vi "Find Unique Zero.vi"(7 "VI in":refnum<vi>, 8 "Error In":errorcluster, 9 "Zero Finder Parameters":T1, 10 "max tau":dbl, 11 "Zeros":dbl[](array[numeric])) -> (0 "Error Out":errorcluster, 3 "Phase Lifetime":dbl)   [LabVIEW 2019]
uses:
  tau_phi & tau_m Zero Finder Parameters.ctl
  <vilib>/gmath/NI_Gmath.lvlib
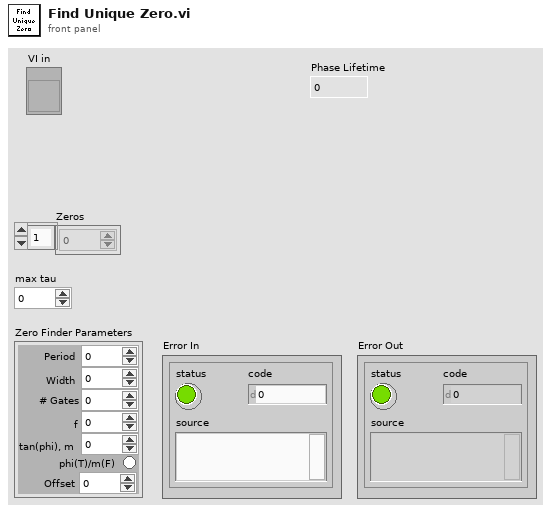
[diagram p1: front panel]
types:
  T1 = typedef "tau_phi & tau_m Zero Finder Parameters.ctl" = cluster{"Period":ext, "Width":ext, "# Gates":ext, "f":ext, "tan(phi), m":ext, "phi(T)/m(F)":bool, "Offset":ext}
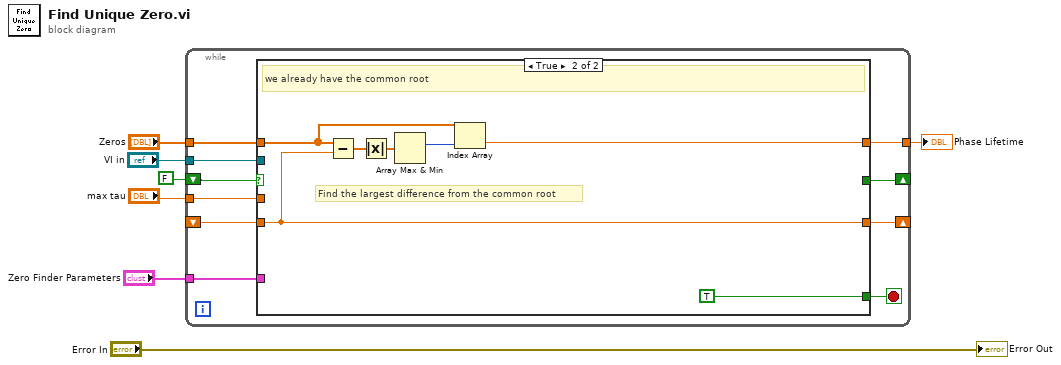
[diagram p0: block diagram]
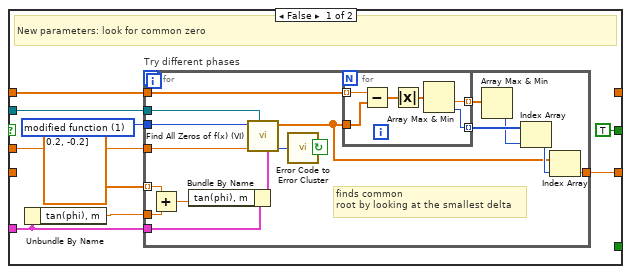
[diagram p2: hidden frame]
diagram:
  n1 = while {
    tunnel: "Zero Finder Parameters" -> [w13]
    shift-right: [w14] -> _
    shift-left: _ -> [w16]
    tunnel: "Zeros" -> [w17]
    tunnel: [w15] -> w4
    tunnel: "VI in" -> [w12]
    tunnel: "max tau" -> [w11]
    shift-right: [w8] -> _
    shift-left: FALSE -> [w9]
    stop <- w10 stop-if-true
    n2 = case shown="True" w9 {
      tunnel: w17 -> [w20 w51]
      tunnel: w16 -> [_ w55]
      tunnel: [_ w50] -> w15
      tunnel: [w19 w55] -> w14
      tunnel: w13 -> [w21 _]
      tunnel: w12 -> [w24 _]
      tunnel: w11 -> [w22 _]
      tunnel: [_ TRUE] -> w10
      tunnel: [TRUE _] -> w8
      frame False {
        w23 = u16 1 items=["fixed function", "modified function"] ("step type")
        # "New parameters: look for common zero"
        n3 = Unbundle By Name(w21) -> ("tan(phi), m"=w26:ext)
        n4 = for "Try different phases" {
          tunnel: w26 -> [w43]
          tunnel: dbl[] [0.1, -0.1, 0.2, -0.2] ("x") -> [w42] mode=indexing
          tunnel: w24 -> [w41]
          tunnel: w23 -> [w40]
          tunnel: w22 -> [w39]
          tunnel: w21 -> [w38]
          tunnel: w20 -> [w33]
          tunnel: [w27] -> w19
          stop <- w34 continue-if-true
          # "finds common\nroot by looking at the smallest delta"
          n5 = Add(x=w42, y=w43) -> (x+y=w36:ext)
          n6 = Bundle By Name(cluster=w38, "tan(phi), m"=w36) -> (w37:T1)
          n7 = call <vilib>:"Find All Zeros of f(x) (VI).vi"("data"=w37, "f(x)"=w41, "end"=w39, "step type"=w40) -> ("error"=w35:i32, "Zeros"=w28:dbl[])  [unwired: 4 in, 2 out]
          n8 = call "Error Code to Error Cluster.vi"("Error Code"=w35) -> ("Error Out"=w34:errorcluster)
          n9 = for {
            tunnel: w33 -> [w49] mode=indexing
            tunnel: w28 -> [w48]
            tunnel: [w45] -> w32 mode=indexing
            tunnel: [w44] -> w31 mode=indexing
            n10 = Subtract(x=w49, y=w48) -> (x-y=w47:dbl[])
            n11 = Absolute Value(x=w47) -> (abs(x)=w46:dbl[])
            n12 = Array Max & Min(array=w46) -> (min value=w45:dbl, min index (indices)=w44:i32)  [unwired: 2 out]
          }
          n13 = Array Max & Min(array=w32) -> (min index (indices)=w30:i32)  [unwired: 3 out]
          n14 = Index Array(array=w31, index=w30) -> (element=w29:i32)
          n15 = Index Array(array=w28, index=w29) -> (element=w27:dbl)
        }
      }
      frame True {
        # "Find the largest difference from the common root"
        # "we already have the common root"
        n16 = Subtract(x=w51, y=w55) -> (x-y=w54:dbl[])
        n17 = Absolute Value(x=w54) -> (abs(x)=w53:dbl[])
        n18 = Array Max & Min(array=w53) -> (max index (indices)=w52:i32)  [unwired: 3 out]
        n19 = Index Array(array=w51, index=w52) -> (element=w50:dbl)
      }
    }
  }
  "Phase Lifetime" <- w4
  "Error Out" <- "Error In"
